vi "Timer.vi"(10 "Enum":enum16{"Start", "Stop"}(ring)) -> (2 "Numeric":u32)   [LabVIEW 2013]
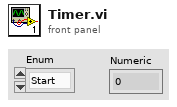
[diagram p1: front panel]
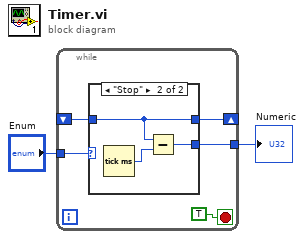
[diagram p0: block diagram]
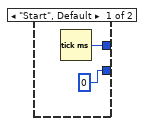
[diagram p2: hidden frame]
diagram:
  n1 = while {
    shift-right: [w3] -> _
    shift-left: _ -> [w5]
    tunnel: "Enum" -> [w6]
    tunnel: [w4] -> w1
    stop <- TRUE stop-if-true
    n2 = case shown="\"Stop\"" w6 {
      tunnel: w5 -> [_ w11]
      tunnel: [u32 0 w12] -> w4
      tunnel: [w8 w11] -> w3
      frame "Start", Default {
        n3 = Tick Count (ms)() -> (millisecond timer value=w8:u32)
      }
      frame "Stop" {
        n4 = Tick Count (ms)() -> (millisecond timer value=w10:u32)
        n5 = Subtract(x=w11, y=w10) -> (x-y=w12:u32)
      }
    }
  }
  "Numeric" <- w1
